vi "Do.vi"(8 "error in (no error)":errorcluster, 10 "Actor in":refnum<class "Actor.lvclass">, 11 "Configure Relays Msg":refnum<class "Configure Relays Msg.lvclass">) -> (0 "error out":errorcluster, 2 "Actor out":refnum<class "Actor.lvclass">)   [LabVIEW 2013, in "LS218.lvlib" / "Configure Relays Msg.lvclass"]
doc: "This VI delivers the message to the actor by calling the appropriate method(s) on the actor."
uses:
  Configure Relays Msg.lvclass
  <vilib>/ActorFramework/Actor/Actor.lvclass
  LS218/LS218.lvclass
  Configure Relays Msg.lvclass/Configure Relays Msg.ctl
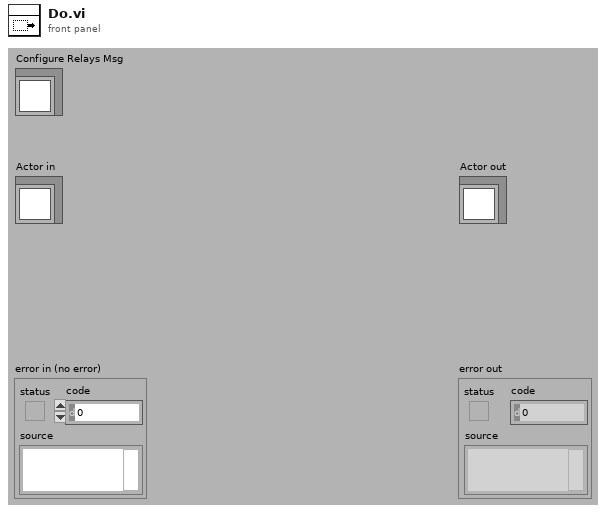
[diagram p1: front panel]
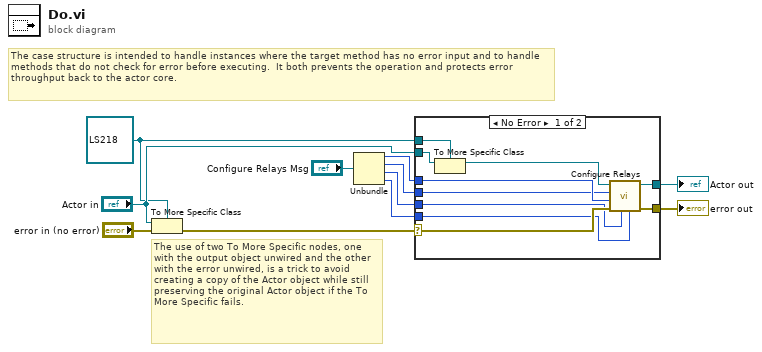
[diagram p0: block diagram]
diagram:
  w5 = refnum<class "LS218.lvclass"> refnum ("Actor in")
  # "The use of two To More Specific nodes, one with the output object unwired and the other with the error unwired, is a trick to avoid creating a copy of the Actor object while still preserving the original Actor object if the To More Specific fails."
  # "The case structure is intended to handle instances where the target method has no error input and to handle methods that do not check for error before executing.  It both prevents the operation and protects error throughput back to the actor core."
  n1 = To More Specific Class(target class=w5, reference="Actor in", error in="error in (no error)") -> (error out=w9:errorcluster)  [unwired: 1 out]
  n2 = Unbundle("Configure Relays Msg") -> (w4:i32, w3:i32, w2:enum16{"Off", "On", "Alarms"}, w1:u16)
  n3 = case shown="No Error" w9 {
    selector: w9 -> [w19 w23]
    tunnel: [w21 w23] -> w8
    tunnel: [w20 w22] -> w7
    tunnel: "Actor in" -> [w18 w22]
    tunnel: w5 -> [w17 _]
    tunnel: w4 -> [w15 _]
    tunnel: w3 -> [w14 _]
    tunnel: w2 -> [w13 _]
    tunnel: w1 -> [w12 _]
    frame No Error {
      n4 = To More Specific Class(target class=w17, reference=w18) -> (specific class reference=w16:refnum<class "LS218.lvclass">)  [unwired: 1 in, 1 out]
      n5 = call "Configure Relays.vi"("Alarm Type (0:Low)"=w12, "Mode (0:Off)"=w13, "error in (no error)"=w19, "Input (0)"=w15, "Relay (0)"=w14, "LS218 in"=w16) -> ("error out"=w21:errorcluster, "LS218 out"=w20:refnum<class "LS218.lvclass">)  [unwired: 4 in]
    }
    frame Error {
      # "If type check fails, pass the original object out again."
    }
  }
  "error out" <- w8
  "Actor out" <- w7
